vi "Feed For Time.vi"(0 "Lower Setpoint":dbl, 1 "Upper Setpoint":dbl, 2 "Duration (s)":dbl, 3 "Command Info In":T1, 4 "Synchronization":enum16{"Start", "Wait"}(ring), 5 "Description":string) -> (10 "Command Info Out":T1)   [LabVIEW 2019]
doc: "This template has a parameter to control whether it waits for the command to complete or not. This is useful for operations that have a timed duration or a sensor-based duration. \n\nBe sure to right-click and select New from Template and save with a new command name."
uses:
  <vilib>/Rock Robotics/WPI/Framework/Command Status Info.ctl
  <vilib>/Rock Robotics/WPI/Framework/Completion Status.ctl
  <vilib>/Rock Robotics/WPI/Framework/Completion Notifier.ctl
  Implementation/Feed Setpoints.ctl
  Implementation/Feed Operations.ctl
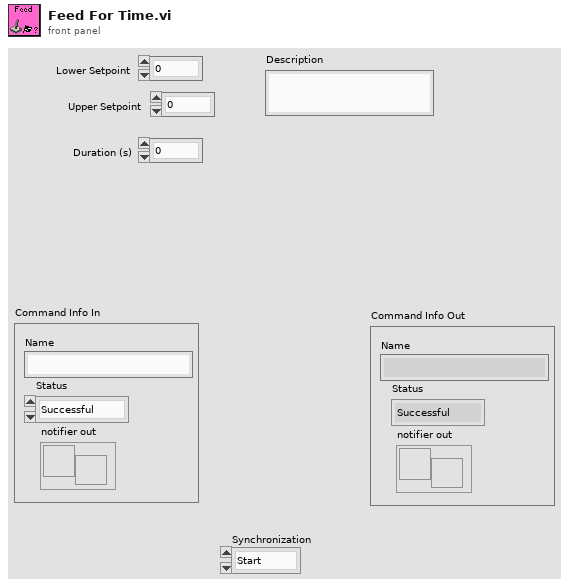
[diagram p1: front panel]
types:
  T1 = typedef "Command Status Info.ctl" = cluster{"Name":string, "Status":T2, "notifier out":T3}
  T2 = typedef "Completion Status.ctl" = enum16{"Successful", "Aborted", "Incomplete"}
  T3 = typedef "Completion Notifier.ctl" = refnum<notifier>
  T4 = typedef "Feed Setpoints.ctl" = cluster{"Operation":T5, "Lower Setpoint":dbl, "Upper Setpoint":dbl, "Duration":dbl}
  T5 = typedef "Feed Operations.ctl" = enum16{"Reserve", "Read Current", "Immediate", "Feed For Time"}
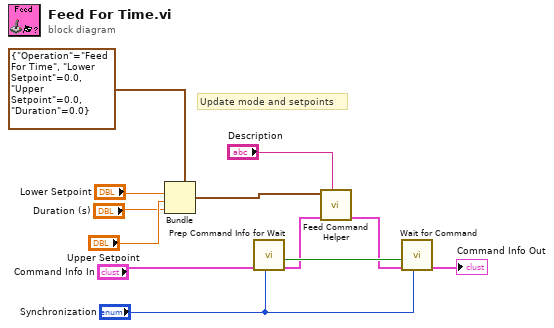
[diagram p0: block diagram]
diagram:
  # "Update mode and setpoints"
  n1 = Bundle(cluster=T4 {"Operation"=enum."Feed For Time", "Lower Setpoint"=0.0, "Upper Setpoint"=0.0, "Duration"=0.0} ("SubSystem Data"), "Lower Setpoint"="Lower Setpoint", "Upper Setpoint"="Upper Setpoint", "Duration"="Duration (s)") -> (w4:T4)  [unwired: 1 in]
  n2 = call <vilib>:"Prep Command Info for Wait.vi"("Synchronication"="Synchronization", "Command Info"="Command Info In") -> ("Command Info"=w8:T1, "Allocated"=w9:bool)  [unwired: 8 in]
  n3 = call "Feed Command Helper.vi"("Description"="Description", "Command Info In"=w8, "SubSystem Data"=w4) -> ("Command Info Out"=w5:T1)  [unwired: 6 in, 2 out]
  n4 = call <vilib>:"Wait for Command.vi"("Synchronication"="Synchronization", "Command Info in"=w5, "Allocated"=w9) -> ("Command Info out"=→"Command Info Out":T1)  [unwired: 8 in]
